vi "Host Main.vi"() -> ()   [LabVIEW 2017]
doc: "This application launches and executes the Tag Bus Data framework configuration for the specified target alias. This is a simple example of the framework API functions, but may also be a suitable starting point for a Host UI or Thick Client that is running a local version of the framework."
uses:
  Utilities/Controlword_Commands.ctl
  Utilities/StateMachine.ctl
  Utilities/Parameters_Reference.ctl
  Utilities/Results_Trajectory.ctl
  Utilities/Results_MotionIO.ctl
  Utilities/Results_Faults.ctl
  <vilib>/NI/STM/TCP/TCP Read Options.ctl
  <vilib>/NI/STM/TCP/Read Meta Data (TCP Ref).vi
  <vilib>/NI/STM/TCP/Get Connection Reference (TCP).vi
  <vilib>/NI/STM/TCP/Read Meta Data (TCP Clst).vi
  <vilib>/NI/STM/Connection Manager/TCP/TCP Connection Manager.vi
  <vilib>/NI/STM/TCP/Write Message (TCP).vi
  <vilib>/NI/STM/TCP/Read Message (TCP).vi
  <vilib>/NI/STM/NI STM.lvlib
  Utilities/WordManipulationLibrary.lvlib
  Utilities/Bit Manipulation.lvlib
panel:
  out "bit value":bool
  in  "Tab Control":T1(tab)
  out "error  out":errorcluster
  in  "Network Stop":bool
  in  "Target IP Address":string="10.1.128.134"
  in  "Results to get":bool
  out "Velocity_Result":dbl
  out "Position_Result":dbl[](array[numeric])
  out "Motion I/O":T2[](array[typedef])
  out "Feedback":T3[](array[typedef])
  out "Fault Data":T4[](array[typedef])
  in  "StateName":string="StateChange"
  in  "Device Control Command":T5
  in  "StateChange":bool
  in  "StraightLineMove":bool
  in  "Acceleration Jerk":dbl=10.0
  in  "Acceleration":dbl=10.0
  in  "Velocity":dbl=10.0
  in  "Positions":dbl[](array[numeric])=[50.0]
  in  "Velocity Move":bool
  in  "Reference Move":bool
  in  "Reference Move Parameters":T6={"Reference Move Mode"=11599899, "Start Search Forward"=FALSE, "Stop on FWD Edge"=FALSE, "Approach Forward"=FALSE, "Velocity"=10.0, "Acceleration"=10.0} {"Reference Move Mode" items=["Home"=11599899, "Index"=11599900, "Center"=11599901, "Forward Limit"=11599902, "Reverse Limit"=11599903, "Absolute"=12648450]}
  out "Raw results":dbl[](array[numeric])
  out "Status":T7
  # "Fast Read"
  # "Full Read"
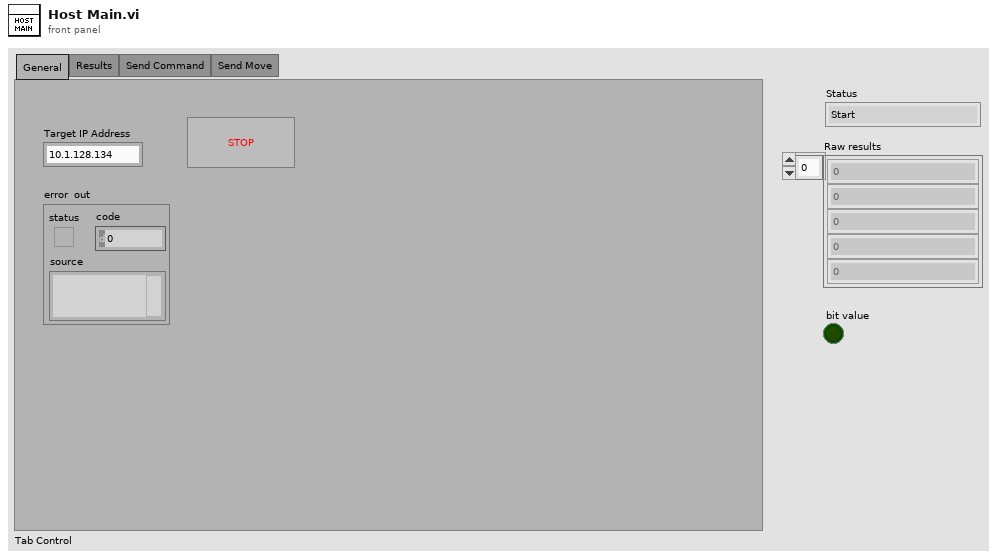
[diagram p1: front panel]
types:
  T1 = enum32{"General", "Results", "Send Command", "Send Move"}
  T2 = typedef "WordManipulationLibrary.lvlib/Results_MotionIO.ctl" = cluster{"Forward Limit Active":bool, "Rev Limit Active":bool, "Home Limit Active":bool, "Forward SW Limit Active":bool, "Rev SW Limit Active":bool, "Drive Fault Active":bool, "Drive Ready":bool, "Target reached Active":bool}
  T3 = typedef "WordManipulationLibrary.lvlib/Results_Trajectory.ctl" = cluster{"Position Setpoint":dbl, "Position Feedback":dbl, "Velocity Setpoint":dbl, "Velocity Feedback":dbl}
  T4 = typedef "WordManipulationLibrary.lvlib/Results_Faults.ctl" = cluster{"Checked Fault":bool, "Fault Code":i32}
  T5 = typedef "WordManipulationLibrary.lvlib/Controlword_Commands.ctl" = enum16{"Shutdown", "Switch On", "Disable Voltage", "Quick Stop", "Disable Op", "Enable Op", "Fault Reset", "Error"}
  T6 = typedef "WordManipulationLibrary.lvlib/Parameters_Reference.ctl" = cluster{"Reference Move Mode":i32, "Start Search Forward":bool, "Stop on FWD Edge":bool, "Approach Forward":bool, "Velocity":dbl, "Acceleration":dbl}
  T7 = typedef "WordManipulationLibrary.lvlib/StateMachine.ctl" = enum16{"Start", "Not Ready to Switch On", "Switch On Disabled", "Ready to Switch On", "Switched On", "Operation enable", "Quick Stop Active", "Fault Reaction Active", "Fault"}
  T8 = typedef "NI STM.lvlib/TCP Read Options.ctl" = cluster{"ignore timeout error":bool, "timeout ms (1000)":i32}
  T9 = typedef "NI STM.lvlib/TCP Connection Info.ctl" = cluster{"connection ID":refnum<k5>, "meta data":T10[]}
  T10 = typedef "NI STM.lvlib/MetaDataElement.ctl" = string
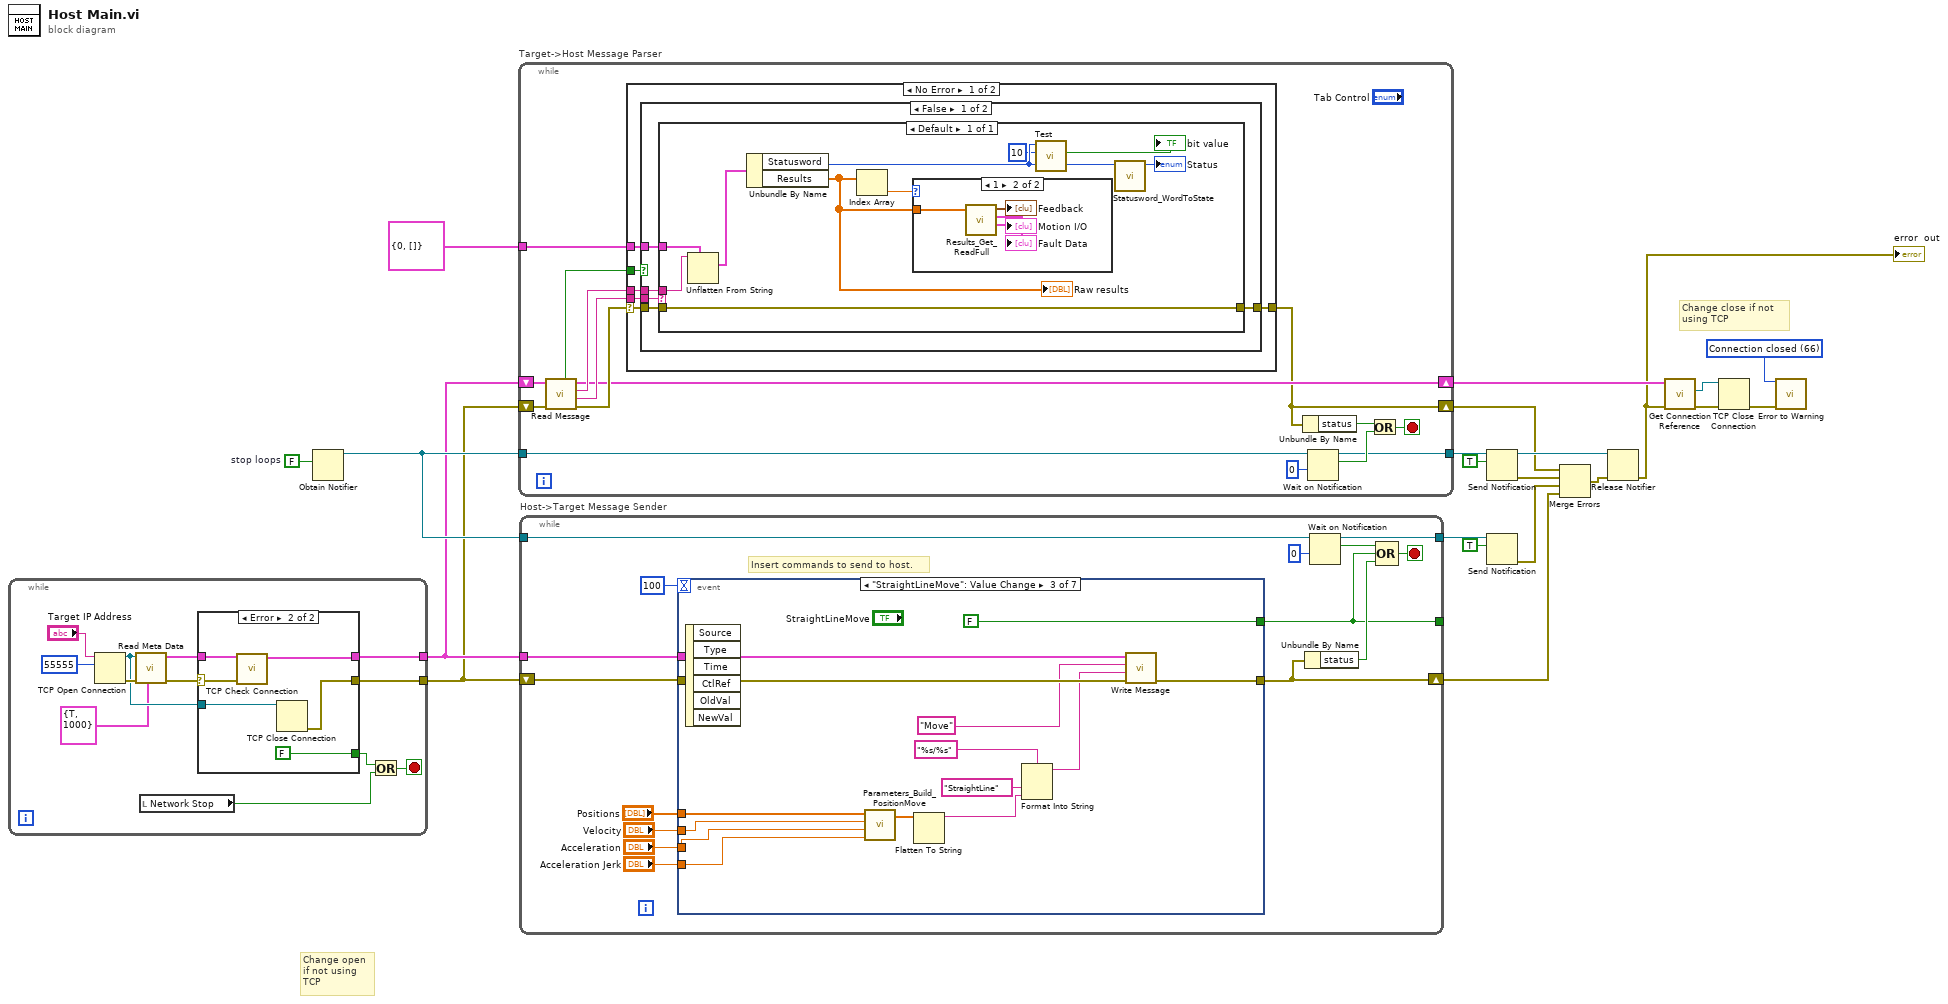
[diagram p0: block diagram]
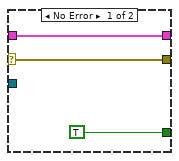
[diagram p2: hidden frame]
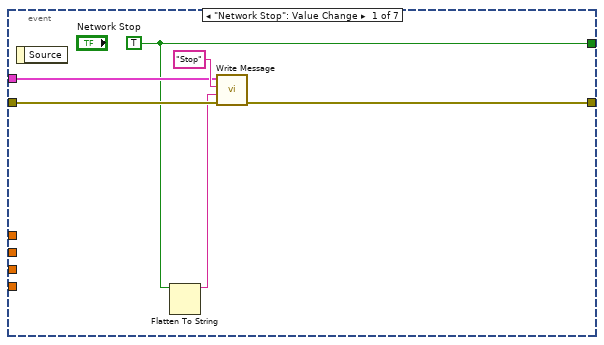
[diagram p3: hidden frame]
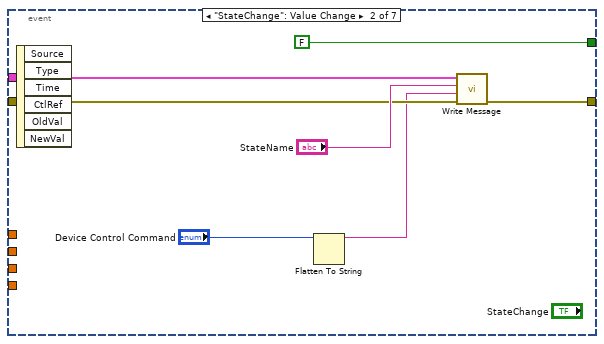
[diagram p4: hidden frame]
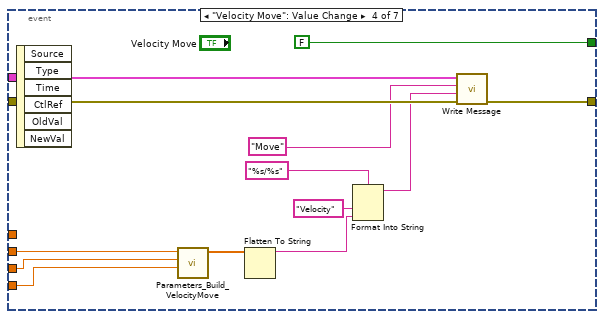
[diagram p5: hidden frame]
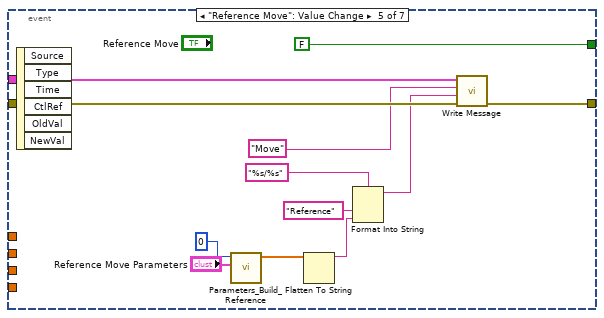
[diagram p6: hidden frame]
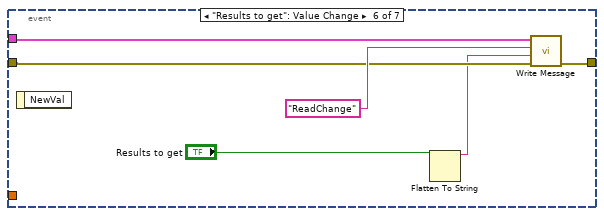
[diagram p7: hidden frame]
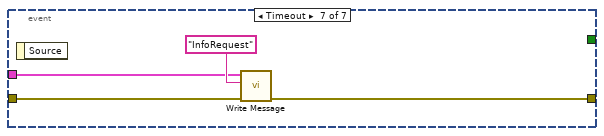
[diagram p8: hidden frame]
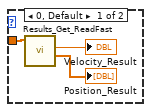
[diagram p9: hidden frame]
diagram:
  w6 = FALSE  # stop loops
  w20 = 66 items=["No Error", "Argument Error", "Memory Full", "Out of Zone", "End of File", "File Already Open", "Generic File IO Error", "File Not Found", "File Permission Error", "Disk Full", "Duplicate Path", "Too Many Files Open", "Not Enabled", "Resource File Not Found", "Cannot Add Resource", "Resource Not Found", "Image Not Found", "Image Memory Error", "Pen Does Not Exist", "Config Bad Type", "Config Token Not Found", "Config Parse Error", "Config Memory Error", "Bad External Code Format", "Bad External Code Offset", "External Code Not Present", "Null Window", "Destroy Window Mixup", "Null Menu", "Print Aborted", "Bad Print Record", "Print Driver Error", "Windows Error During Print", "Memory Error During Print", "Print Dialog Error", "Generic Print Error", "Invalid Device Refnum", "Device Not Found", "Device Parameter Error", "Device Unit Error", "Can't Open Device", "Device Call Aborted", "Generic Error", "Cancelled By User", "Object ID Too Low", "Object ID Too High", "Object Not In Heap", "Unknown Heap", "Bad DefProc ID", "DefProc Not In Table", "Message Out Of Range", "Null Method", "Unknown Message", "Manager Call Not Supported", "Bad address", "Connection In progress", "Connection timed out", "Connection is already in progress", "Network attribute not supported", "Network error", "Address in use", "System out of memory", "Connection aborted", "Connection refused", "Connection is not connected", "Connection is already connected", "Connection closed", "Initialize error (interapplication manager)", "Bad occurrence", "Wait on unbound occurrence handler", "Occurrence queue overflow", "Bad path", "Semaphore not signaled", "Unrecognized type (interapplication manager)"] ("1st Error to Convert")
  # "Change close if not using TCP"
  # "Change open if not using TCP"
  n1 = while {
    tunnel: [w29] -> w5
    tunnel: [w27] -> w4
    stop <- w24 stop-if-true
    n2 = TCP Open Connection(address="Target IP Address", remote port or service name=u16 55555 ("remote port")) -> (connection ID=w26:refnum<k5>, error out=w33:errorcluster)  [unwired: 1 in, 2 out]
    n3 = call-poly <vilib>:"Read Meta Data.vi"("options"=T8 {"ignore timeout error"=TRUE, "timeout ms (1000)"=1000}, "error in"=w33, "connection ID"=w26) -> ("error out"=w30:errorcluster, "connection info out"=w28:T9)  [unwired: 7 out]
    n4 = local read "Network Stop"() -> (w23:bool)
    n5 = case shown="Error" w30 {
      selector: w30 -> [w34 w40]
      tunnel: [TRUE FALSE] -> w25
      tunnel: [w35 w39] -> w29
      tunnel: w28 -> [w35 w41]
      tunnel: [w34 w37] -> w27
      tunnel: w26 -> [_ w42]
      frame No Error {
      }
      frame Error {
        n6 = call <vilib>:"TCP Check Connection.vi"("error in"=w40, "connection in"=w41) -> ("connection out"=w39:T9)  [unwired: 7 in, 2 out]
        n7 = TCP Close Connection(connection ID=w42) -> (error out=w37:errorcluster)  [unwired: 2 in, 1 out]
      }
    }
    n8 = Or(x=w25, y=w23) -> (x .or. y?=w24:bool)
  }
  n9 = Obtain Notifier(notification data type=w6) -> (notifier out=w9:refnum<notifier>)  [unwired: 3 in, 2 out]
  n10 = while "Target->Host Message Parser" {
    shift-right: [w44] -> w3
    shift-left: w4 -> [w56]
    tunnel: w9 -> [w50]
    tunnel: [w46] -> w7
    shift-right: [w51] -> w19
    shift-left: w5 -> [w57]
    tunnel: cluster{"Statusword":u16, "Results":dbl[]} {"Statusword"=0, "Results"=[]} ("Parameters to process") -> [w43]
    stop <- w47 stop-if-true
    n11 = call-poly <vilib>:"Read Message.vi"("error in"=w56, "connection info in"=w57) -> ("error out"=w52:errorcluster, "name"=w55:T10, "data string"=w54:string, "connection info out"=w51:T9, "timed out?"=w53:bool)  [unwired: 3 in, 2 out]
    n12 = case shown="No Error" w52 {
      selector: w52 -> [w60 w87]
      tunnel: w55 -> [w63 _]
      tunnel: w54 -> [w62 _]
      tunnel: w53 -> [w61 _]
      tunnel: [w59 w87] -> w44
      tunnel: w43 -> [w58 _]
      frame No Error {
        n13 = case shown="False" w61 {
          tunnel: w63 -> [w65 _]
          tunnel: w62 -> [w68 _]
          tunnel: w60 -> [w67 w86]
          tunnel: [w66 w86] -> w59
          tunnel: w58 -> [w64 _]
          frame False {
            n14 = case shown="Default" w65 {
              tunnel: w68 -> [w77]
              tunnel: w67 -> [w78]
              tunnel: [w78] -> w66
              tunnel: w64 -> [w76]
              frame Default {
                n15 = Unflatten From String(type=w76, binary string=w77) -> (value=w75:cluster{"Statusword":u16, "Results":dbl[]})  [unwired: 3 in, 2 out]
                n16 = Unbundle By Name(w75) -> ("Statusword"=w71:u16, "Results"=w72:dbl[])
                "Raw results" <- w72
                n17 = Index Array(array=w72) -> (element=w73:dbl)  [unwired: 1 in]
                n18 = case shown="1" w73 {
                  tunnel: w72 -> [w81 w85]
                  frame 0, Default {
                    n19 = call "Results_Get_ReadFast.vi"("Results"=w81) -> ("Position"=→"Position_Result":dbl[], "Velocity"=→"Velocity_Result":dbl)  [unwired: 9 in]
                  }
                  frame 1 {
                    n20 = call "Results_Get_ReadFull.vi"("appended array"=w85) -> ("Fault Data"=→"Fault Data":T4[], "Motion I/O"=→"Motion I/O":T2[], "Feedback"=→"Feedback":T3[])  [unwired: 7 in, 1 out]
                  }
                }
                n21 = call "Test.vi"("Bit to test"=u8 10, "Data_In"=w71) -> ("bit value"=→"bit value":bool)  [unwired: 8 in, 1 out]
                n22 = call "Statusword_WordToState.vi"("Data_In"=w71) -> ("Status"=→"Status":T7)  [unwired: 10 in]
              }
            }
          }
          frame True {
          }
        }
      }
      frame Error {
      }
    }
    n23 = Unbundle By Name(w44) -> ("status"=w45:bool)
    n24 = Wait on Notification(notifier=w50, timeout in ms (-1)=0) -> (notifier out=w46:refnum<notifier>, notification=w48:bool)  [unwired: 2 in, 2 out]
    n25 = Or(x=w45, y=w48) -> (x .or. y?=w47:bool)
  }
  n26 = while "Host->Target Message Sender" {
    shift-right: [w94] -> w12
    shift-left: w4 -> [w102]
    tunnel: w5 -> [w101]
    tunnel: w9 -> [w98]
    tunnel: [w95] -> w10
    tunnel: [w92] -> _
    stop <- w96 stop-if-true
    # "Insert commands to send to host."
    n27 = event shown="[2] \"StraightLineMove\": Value Change" {
      selector: _ -> [_ _ _ _ _ _ _]
      dyn-events: _ -> [_ _ _ _ _ _ _]
      timeout: 100 -> [_ _ _ _ _ _ _]
      tunnel: w101 -> [w107 w114 w129 w142 w154 w159 w161]
      tunnel: w102 -> [w106 w113 w128 w141 w153 w158 w164]
      tunnel: [w104 FALSE ("stop") FALSE ("stop") FALSE ("stop") FALSE ("stop") _ _] -> w92
      tunnel: [w103 w110 w126 w139 w151 w157 w163] -> w94
      tunnel: "Positions" -> [_ _ w119 _ _ _ _]
      tunnel: "Velocity" -> [_ _ w118 w133 _ _ _]
      tunnel: "Acceleration" -> [_ _ w117 w131 _ _ _]
      tunnel: "Acceleration Jerk" -> [_ _ w116 w130 _ _ _]
      event "Network Stop": Value Change {
        w104 = TRUE ("stop")
        n28 = event-data() -> ()  [unwired: 2 out]
        n29 = Flatten To String(anything=w104) -> (data string=w105:string)  [unwired: 2 in, 3 out]
        n30 = call-poly <vilib>:"Write Message.vi"("error in"=w106, "data"=w105, "name"="Stop" ("Name"), "connection info in"=w107) -> ("error out"=w103:errorcluster)  [unwired: 1 in, 6 out]
      }
      event "StateChange": Value Change {
        n31 = event-data() -> ()  [unwired: 7 out]
        n32 = Flatten To String(anything="Device Control Command") -> (data string=w112:string)  [unwired: 2 in, 3 out]
        n33 = call-poly <vilib>:"Write Message.vi"("error in"=w113, "data"=w112, "name"="StateName", "connection info in"=w114) -> ("error out"=w110:errorcluster)  [unwired: 1 in, 6 out]
      }
      event "StraightLineMove": Value Change {
        n34 = event-data() -> ()  [unwired: 7 out]
        n35 = call "Parameters_Build_PositionMove.vi"("Acceleration Jerk"=w116, "Acceleration"=w117, "Velocity"=w118, "Positions"=w119) -> ("Parameters"=w121:dbl[])  [unwired: 7 in]
        n36 = Flatten To String(anything=w121) -> (data string=w120:string)  [unwired: 2 in, 3 out]
        n37 = Format Into String(format string="%s/%s", "StraightLine" ("input 1"), w120) -> (resulting string=w122:string)  [unwired: 2 in, 1 out]
        n38 = call-poly <vilib>:"Write Message.vi"("error in"=w128, "data"=w122, "name"="Move", "connection info in"=w129) -> ("error out"=w126:errorcluster)  [unwired: 1 in, 6 out]
      }
      event "Velocity Move": Value Change {
        n39 = event-data() -> ()  [unwired: 7 out]
        n40 = call "Parameters_Build_VelocityMove.vi"("Acceleration Jerk"=w130, "Acceleration"=w131, "Velocity"=w133) -> ("Parameters"=w132:dbl[])  [unwired: 8 in]
        n41 = Flatten To String(anything=w132) -> (data string=w134:string)  [unwired: 2 in, 3 out]
        n42 = Format Into String(format string="%s/%s", "Velocity" ("input 1"), w134) -> (resulting string=w135:string)  [unwired: 2 in, 1 out]
        n43 = call-poly <vilib>:"Write Message.vi"("error in"=w141, "data"=w135, "name"="Move", "connection info in"=w142) -> ("error out"=w139:errorcluster)  [unwired: 1 in, 6 out]
      }
      event "Reference Move": Value Change {
        n44 = event-data() -> ()  [unwired: 7 out]
        n45 = call "Parameters_Build_Reference.vi"("Reference Move Parameters"="Reference Move Parameters", "Axis to command"=0) -> ("Parameters"=w144:dbl[])  [unwired: 9 in]
        n46 = Flatten To String(anything=w144) -> (data string=w143:string)  [unwired: 2 in, 3 out]
        n47 = Format Into String(format string="%s/%s", "Reference" ("input 1"), w143) -> (resulting string=w147:string)  [unwired: 2 in, 1 out]
        n48 = call-poly <vilib>:"Write Message.vi"("error in"=w153, "data"=w147, "name"="Move", "connection info in"=w154) -> ("error out"=w151:errorcluster)  [unwired: 1 in, 6 out]
      }
      event "Results to get": Value Change {
        n49 = event-data() -> ()  [unwired: 2 out]
        n50 = Flatten To String(anything="Results to get") -> (data string=w156:string)  [unwired: 3 in, 2 out]
        n51 = call-poly <vilib>:"Write Message.vi"("error in"=w158, "data"=w156, "name"="ReadChange", "connection info in"=w159) -> ("error out"=w157:errorcluster)  [unwired: 1 in, 6 out]
      }
      event Timeout {
        n52 = event-data() -> ()  [unwired: 2 out]
        n53 = call-poly <vilib>:"Write Message.vi"("error in"=w164, "name"="InfoRequest", "connection info in"=w161) -> ("error out"=w163:errorcluster)  [unwired: 7 in, 1 out]
      }
    }
    n54 = Unbundle By Name(w94) -> ("status"=w93:bool)
    n55 = Wait on Notification(notifier=w98, timeout in ms (-1)=0) -> (notifier out=w95:refnum<notifier>, notification=w100:bool)  [unwired: 2 in, 2 out]
    n56 = Compound Arithmetic op=OR(w100, w92, w93) -> (w96:bool)
  }
  n57 = Send Notification(notification=TRUE, notifier=w7) -> (notifier out=w15:refnum<notifier>, error out=w14:errorcluster)  [unwired: 1 in]
  n58 = Send Notification(notification=TRUE, notifier=w10) -> (error out=w13:errorcluster)  [unwired: 1 in, 1 out]
  n59 = Merge Errors(w3, w14, w13, w12) -> (w16:errorcluster)
  n60 = Release Notifier(notifier=w15, error in (no error)=w16) -> (error out=w1:errorcluster)  [unwired: 1 in, 2 out]
  "error  out" <- w1
  n61 = call-poly <vilib>:"Get Connection Reference.vi"("error in"=w1, "connection info in"=w19) -> ("error out"=w18:errorcluster, "connection ID out"=w17:refnum<k5>)  [unwired: 8 out]
  n62 = TCP Close Connection(connection ID=w17, error in (no error)=w18) -> (error out=w21:errorcluster)  [unwired: 2 out]
  n63 = call <vilib>:"Error to Warning.vi"("1st Error to Convert"=w20, "error in"=w21) -> ()  [unwired: 3 in, 11 out]
